vi "Set Default.vi"   [LabVIEW 2018]
uses:
  <vilib>/rvi/eio/common/nirviEmuTemplateMethod_errors.vi
  <vilib>/eio/EIONode/EIONode.xnode
panel:
  # "Initialize default Values for Electronics"
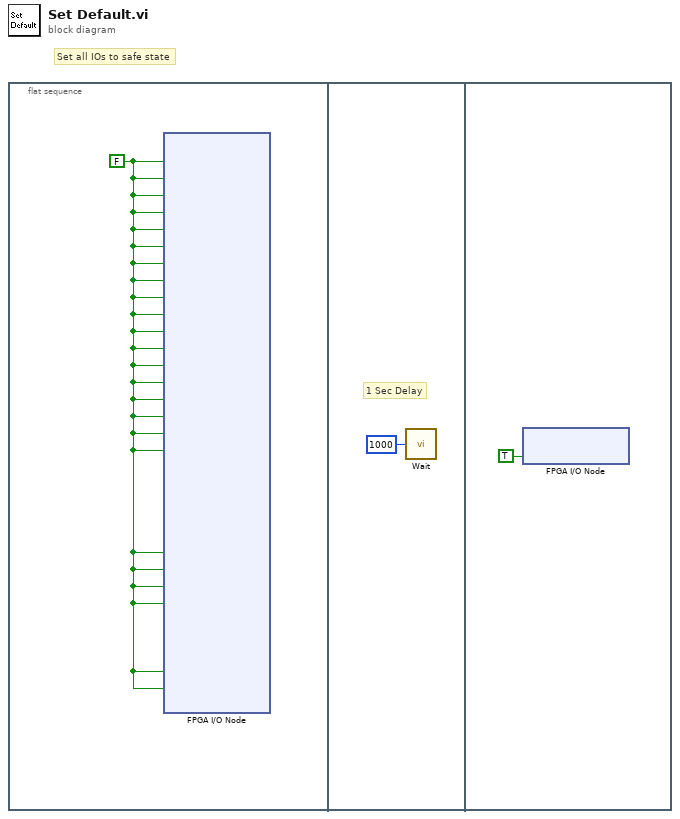
[diagram p0: block diagram]
diagram:
  # "Set all IOs to safe state"
  n1 = flat-sequence {
    frame #0 {
      w1 = FALSE ("RMC/DIO57")
      n2 = xnode "FPGA I/O Node"("D0"=w1, "D1"=w1, "D2"=w1, "D3"=w1, "D4"=w1, "D5"=w1, "D6"=w1, "D7"=w1, "D8"=w1, "D9"=w1, "D10"=w1, "D11"=w1, "D12"=w1, "D13"=w1, "D14"=w1, "D15"=w1, "D16"=w1, "D17"=w1, "RMC/DIO18"=w1, "Electronics"=w1, "RMC/DIO57"=w1, "RMC/DIO58"=w1, "RMC/DIO66"=w1, "RMC/DIO67"=w1) -> ()  [unwired: 33 in, 42 out]
    }
    frame #1 {
      # "1 Sec Delay"
      n3 = call "Wait"("Count(mSec)"=u16 1000) -> ()  [unwired: 1 out]
    }
    frame #2 {
      n4 = xnode "FPGA I/O Node"("RMC/DIO57"=TRUE) -> ()  [unwired: 1 in, 1 out]
    }
  }
